vi "ADT file path.vi"(0 "error in":errorcluster) -> (1 "error out":errorcluster, 2 "dup path":path)   [LabVIEW 2015]
uses:
  <vilib>/Utility/config.llb/NI_LVConfig.lvlib
  <vilib>/Utility/config.llb/Read Key (Boolean).vi
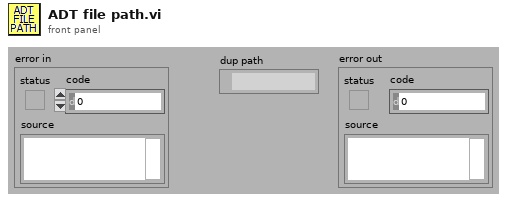
[diagram p1: front panel]
types:
  T1 = typedef "NI_LVConfig.lvlib/Config Data RefNum.ctl" = refnum<k1>
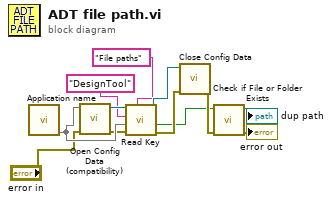
[diagram p0: block diagram]
diagram:
  n1 = call "Application name.vi"() -> (0:w7)  [unwired: 4 in, 3 out]
  n2 = call <vilib>:"Open Config Data (compatibility).vi"("error in (no error)"="error in", "configuration file path"=w7) -> ("error out"=w3:errorcluster, "refnum"=w8:T1)  [unwired: 7 in, 1 out]
  n3 = call-poly <vilib>:"Read Key.vi"("section"="File paths", "error in (no error)"=w3, "default value"=w7, "key"="DesignTool", "refnum"=w8) -> ("error out"=w10:errorcluster, "value"=w2:bool, "refnum out"=w9:T1)  [unwired: 3 in, 1 out]
  n4 = call <vilib>:"Close Config Data.vi"("error in (no error)"=w10, "refnum"=w9) -> ("error out"=w11:errorcluster)  [unwired: 8 in, 1 out]
  n5 = call <vilib>:"Check if File or Folder Exists.vi"("error in (no error)"=w11, "path"=w2) -> ("error out"=→"error out":errorcluster, "dup path"=→"dup path":path)  [unwired: 7 in, 1 out]
